vi "B7_65_ErrorAnswer.vi"(4 "input":u8=1 format="%b") -> (1 "Error answer string":string)   [LabVIEW 2018]
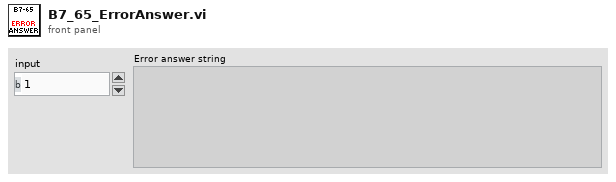
[diagram p1: front panel]
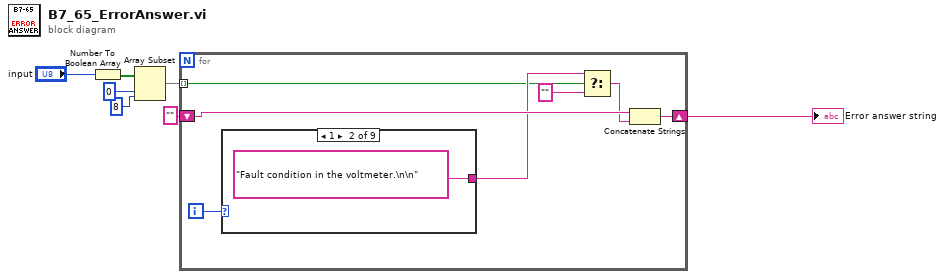
[diagram p0: block diagram]
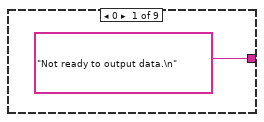
[diagram p2: hidden frame]
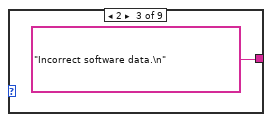
[diagram p3: hidden frame]
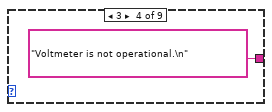
[diagram p4: hidden frame]
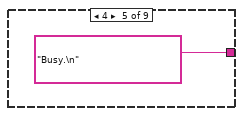
[diagram p5: hidden frame]
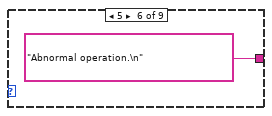
[diagram p6: hidden frame]
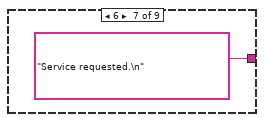
[diagram p7: hidden frame]
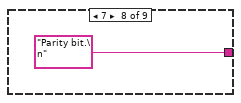
[diagram p8: hidden frame]
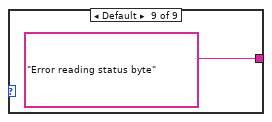
[diagram p9: hidden frame]
diagram:
  n1 = Number To Boolean Array(number="input") -> (Boolean array=w7:bool[])
  n2 = Array Subset(array=w7, index=0, length=8) -> (w4:bool[])
  n3 = for {
    tunnel: w4 -> [w8] mode=indexing
    shift-right: [w12] -> w1
    shift-left: "" ("Driver Name") -> [w13]
    i -> [w14]
    n4 = case shown="1" w14 {
      tunnel: ["Not ready to output data.\n" ("Driver Name") "Fault condition in the voltmeter.\n\n" ("Driver Name") "Incorrect software data.\n" ("Driver Name") "Voltmeter is not operational.\n" ("Driver Name") "Busy.\n" ("Driver Name") "Abnormal operation.\n" ("Driver Name") "Service requested.\n" ("Driver Name") "Parity bit.\n" ("Driver Name") "Error reading status byte" ("Driver Name")] -> w10
      frame 0 {
      }
      frame 1 {
      }
      frame 2 {
      }
      frame 3 {
      }
      frame 4 {
      }
      frame 5 {
      }
      frame 6 {
      }
      frame 7 {
      }
      frame Default {
      }
    }
    n5 = Select(t=w10, s=w8, f="" ("Driver Name")) -> (s? t:f=w11:string)
    n6 = Concatenate Strings(w13, w11) -> (w12:string)
  }
  "Error answer string" <- w1
